vi "test KVP Arrays.vi"(8 "error in (no error)":errorcluster) -> (0 "error out":errorcluster)   [LabVIEW 2013]
uses:
  <vilib>/addons/_JKI Toolkits/Caraya/classes/Assert/Assert Equal Value_Variant.vi
  <vilib>/addons/_JKI Toolkits/Caraya/classes/Test/Test.lvclass
  <vilib>/addons/_JKI Toolkits/Caraya/classes/Assert/Assert.lvclass
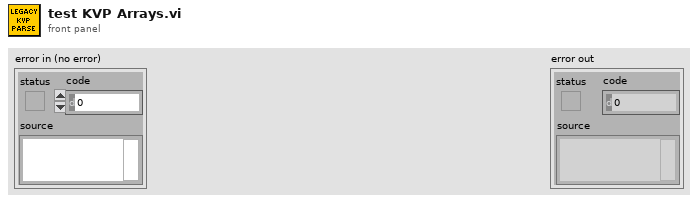
[diagram p1: front panel]
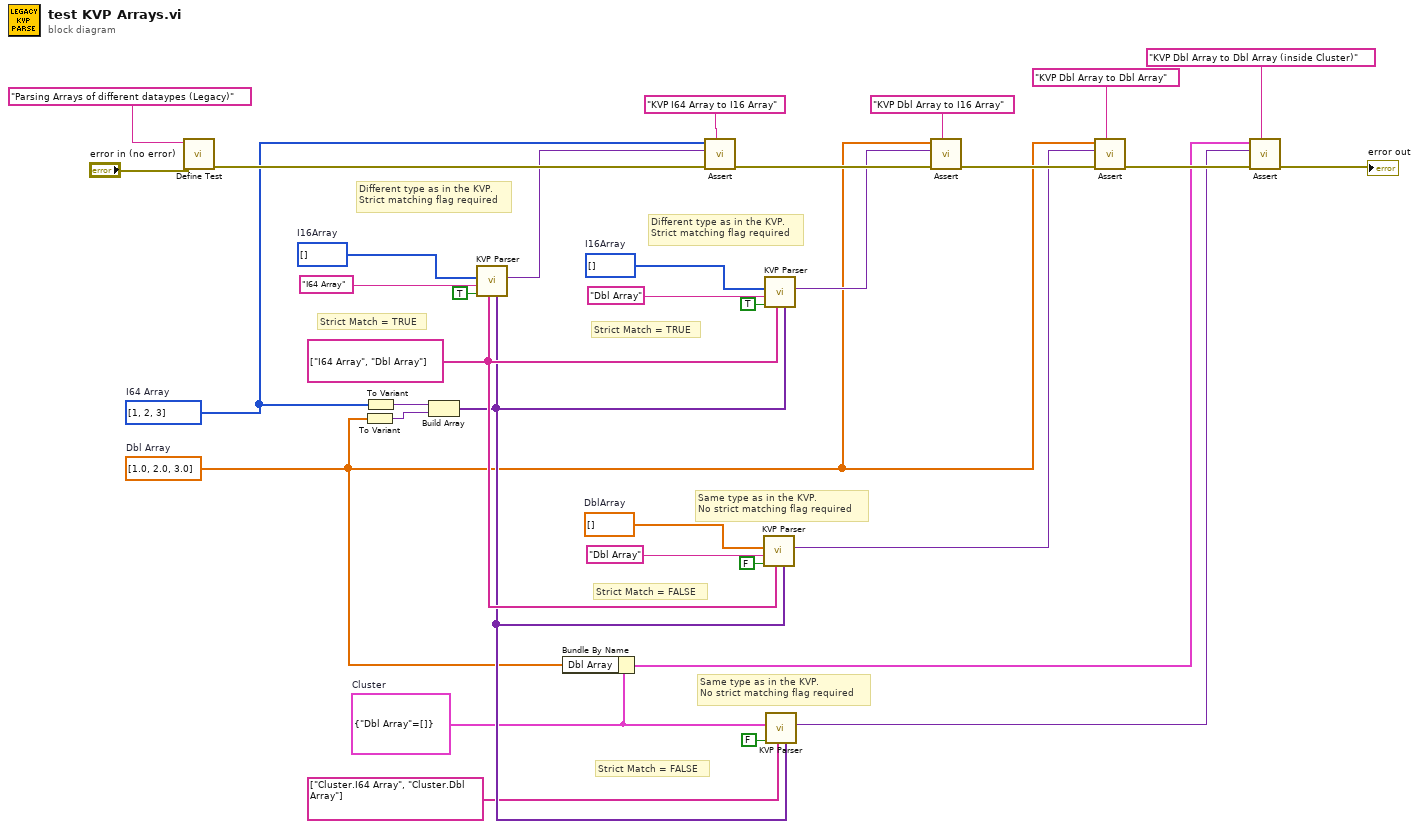
[diagram p0: block diagram]
diagram:
  w5 = cluster{"Dbl Array":dbl[]} {"Dbl Array"=[]}  # Cluster
  w16 = dbl[] []  # DblArray
  w25 = i16[] []  # I16Array
  w4 = dbl[] [1.0, 2.0, 3.0]  # Dbl Array
  w11 = string[] ["I64 Array", "Dbl Array"]
  w28 = i64[] [1, 2, 3]  # I64 Array
  w26 = i16[] []  # I16Array
  # "Same type as in the KVP.\nNo strict matching flag required"
  # "Strict Match = FALSE"
  # "Different type as in the KVP.\nStrict matching flag required"
  # "Different type as in the KVP.\nStrict matching flag required"
  # "Same type as in the KVP.\nNo strict matching flag required"
  # "Strict Match = FALSE"
  # "Strict Match = TRUE"
  # "Strict Match = TRUE"
  n1 = call <vilib>:"Define Test.vi"("error in (no error)"="error in (no error)", "Label (VI Title)"="Parsing Arrays of different dataypes (Legacy)") -> ("error out"=w30:errorcluster)  [unwired: 9 in]
  n2 = To Variant(anything=w4) -> (Variant=w19:variant)
  n3 = To Variant(anything=w28) -> (Variant=w34:variant)
  n4 = Build Array(w34, w19) -> (w10:variant[])
  n5 = call "KVP Parser.vi"("Values"=w10, "Keys"=w11, "Strict type matching? (F)"=TRUE, "Default Value Name (empty: label)"="I64 Array", "Default Value"=w26) -> ("Value"=w29:variant)  [unwired: 3 in, 3 out]
  n6 = Bundle By Name(cluster=w5, "Dbl Array"=w4) -> (w3:cluster{"Dbl Array":dbl[]})
  n7 = call-poly <vilib>:"Assert.vi"("Label"="KVP I64 Array to I16 Array" ("Label (VI Title)"), "error in (no error)"=w30, "Y"=w29, "X"=w28) -> ("error out"=w21:errorcluster)  [unwired: 7 in]
  n8 = call "KVP Parser.vi"("Values"=w10, "Keys"=w11, "Strict type matching? (F)"=FALSE, "Default Value Name (empty: label)"="Dbl Array", "Default Value"=w16) -> ("Value"=w13:variant)  [unwired: 3 in, 3 out]
  n9 = call "KVP Parser.vi"("Values"=w10, "Keys"=w11, "Strict type matching? (F)"=TRUE, "Default Value Name (empty: label)"="Dbl Array", "Default Value"=w25) -> ("Value"=w20:variant)  [unwired: 3 in, 3 out]
  n10 = call "KVP Parser.vi"("Values"=w10, "Keys"=string[] ["Cluster.I64 Array", "Cluster.Dbl Array"], "Strict type matching? (F)"=FALSE, "Default Value"=w5) -> ("Value"=w2:variant)  [unwired: 4 in, 3 out]
  n11 = call-poly <vilib>:"Assert.vi"("Label"="KVP Dbl Array to I16 Array" ("Label (VI Title)"), "error in (no error)"=w21, "Y"=w20, "X"=w4) -> ("error out"=w14:errorcluster)  [unwired: 7 in]
  n12 = call-poly <vilib>:"Assert.vi"("Label"="KVP Dbl Array to Dbl Array" ("Label (VI Title)"), "error in (no error)"=w14, "Y"=w13, "X"=w4) -> ("error out"=w7:errorcluster)  [unwired: 7 in]
  n13 = call-poly <vilib>:"Assert.vi"("Label"="KVP Dbl Array to Dbl Array (inside Cluster)" ("Label (VI Title)"), "error in (no error)"=w7, "Y"=w2, "X"=w3) -> ("error out"=→"error out":errorcluster)  [unwired: 7 in]
